vi "EventLog.CreateError(array).vi"(4 "Level (Error)":T3=enum."Error", 6 "Code (-1)":i32=-1, 7 "Source (All)":T2, 8 "error in":errorcluster, 9 "args":variant[](array[variant]), 10 "Msg":T1, 11 "create (T)":bool=TRUE) -> (0 "error out":errorcluster, 2 "text out":string)   [LabVIEW 2016]
uses:
  EventLog.EventLevel.ctl
  EventLog.EventSource.ctl
  Translator/Translator.Message.ctl
  EventLog.New(array).vi
  Tma.lib/string.llb/Join array to string.vi
  EventLog.File.ReadWrite.vi
  EventLog.Buffer.vi
  Global/ApplicationGlobal.vi
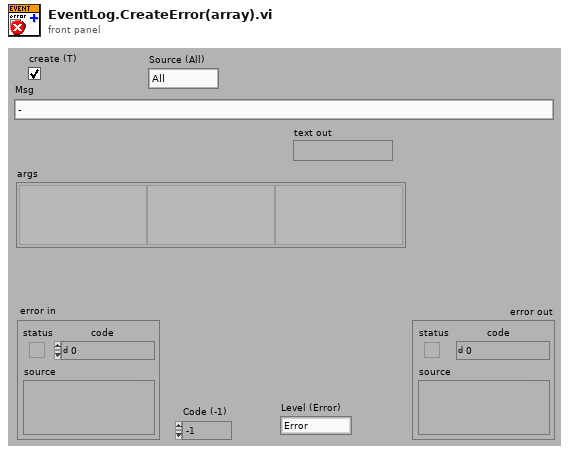
[diagram p1: front panel]
types:
  T1 = typedef "Translator.Message.ctl" = enum16{"-", "Event confirmed", "Log out", "Log in", "Shutdown", "Cancel", "Start", "Continue", "Stop", "On", "Off", "OK", "NOK", "NOK %s", "This", "Prev", "Home", "Work", "In progress...", "Missing", "Empty", "Hardware failure", "Initial", "Error %d >> %s", "Error %d >> %s >> %s", "Starting %s", "Quitting %s", "Configured", "Initializing", "Quitting", "Loading", "Running %s", "Stopped", "Summary", "Do you want to continue?", "Do you want to exit?", "Log out?", "System", "All", "IDLE", "Translating...%s", "Not found", "Alarm %s", "Run", "Skip", "Abort", "Repeat", "Please wait...", "Database disconnected", "Login to database successful", "Login to database failed: %d; %s", "Get process step data for %s", "Changeover off", "Changeover into %s", "Product %s | %s found in cache with status %d at previous station", "Product %s | %s found in database with status %d at previous station", "Product %s | %s not found in cache at previous station", "Product %s | %s not found in database at previous station", "Product %s | %s found in cache with status %d at this station (%d repetion)", "Product %s | %s found in database with status %d at this station (%d repetition)", "Product %s | %s not found in cache at this station", "Product %s | %s not found in database at this station", "Product %s | %s found in cache for component %s | %s", "Product %s | %s found in database for component %s | %s", "Product not found in cache for component %s | %s", "Product not found in database for component %s | %s", "Product %s | %s connected with component %s | %s (cache)", "Product %s | %s connected with component %s | %s (database)", "New data for %s | %s (cache)", "New data for %s | %s (database)", "File %s moved (cache)", "File %s deleted (cache)", "Msg %d >> %s", "PLC LifeBit Failure", "Reconnecting DB", "Reconnecting PLC", "Free disk space is below 1GB - contact technician", "Unable to check product status", "Product %s SN %s checked in DB", "Unable To check status from station %s"}
  T2 = typedef "EventLog.EventSource.ctl" = enum16{"All", "Gui", "Cache", "PLC1", "PLC2", "PLC3", "DB", "DB01", "DB02", "DB03", "DB04", "DB05", "DB06", "DB07", "DB08", "DB09", "DB10", "DB11", "DB12", "DB13", "DB14", "DB15", "DB16"}
  T3 = typedef "EventLog.EventLevel.ctl" = enum8{"Debug", "Info", "Warning", "Error"}
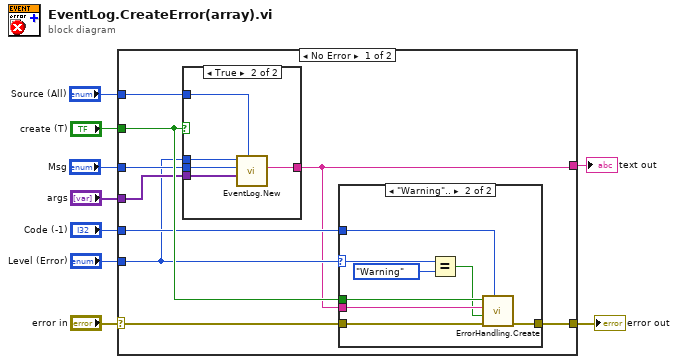
[diagram p0: block diagram]
diagram:
  n1 = case shown="No Error" "error in" {
    selector: "error in" -> [w17 w33]
    tunnel: [w16 w33] -> w9
    tunnel: "create (T)" -> [w18 _]
    tunnel: "Msg" -> [w15 _]
    tunnel: "args" -> [w14 _]
    tunnel: "Code (-1)" -> [w13 _]
    tunnel: "Level (Error)" -> [w12 _]
    tunnel: "Source (All)" -> [w11 _]
    tunnel: [w10 _] -> w2
    frame No Error {
      n2 = case shown="True" w18 {
        tunnel: w15 -> [_ w32]
        tunnel: w14 -> [_ w31]
        tunnel: [_ w30] -> w10
        tunnel: w12 -> [_ w29]
        tunnel: w11 -> [_ w28]
        frame False {
        }
        frame True {
          n3 = call-poly "EventLog.New.vi"("Source (All)"=w28, "Arguments"=w31, "Message (-)"=w32, "Level (Info)"=w29) -> ("Translated Msg"=w30:string)  [unwired: 6 in, 1 out]
        }
      }
      n4 = case shown="\"Warning\".." w12 {
        selector: w12 -> [_ w22]
        tunnel: w18 -> [_ w27]
        tunnel: w17 -> [w19 w26]
        tunnel: [w19 w25] -> w16
        tunnel: w10 -> [_ w24]
        tunnel: w13 -> [_ w23]
        frame Default {
        }
        frame "Warning".. {
          n5 = Equal?(x=w22, y=EventLog.EventLevel."Warning") -> (x = y?=w20:bool)
          n6 = call "ErrorHandling.Create.vi"("error code (5000)"=w23, "error in"=w26, "warning only (F)"=w20, "explanation"=w24, "create (T)"=w27) -> ("error out"=w25:errorcluster)  [unwired: 6 in]
        }
      }
    }
    frame Error {
    }
  }
  "error out" <- w9
  "text out" <- w2
